vi "Create.vi"(7 "options":T13={"FIFO Options"={"Infinite Timeouts"=FALSE}, "Thread Options"={"Show FP On Call"=FALSE, "Close FP After Call"=FALSE, "Allow Debugging"=FALSE}, "Plugin Options"={"Default Components"=FALSE}, "Performance Options"={"Measure Period"=FALSE, "Measure Rx/Tx Duration"=FALSE}, "Data Server Options"={"Enable Data Server"=FALSE, "Period"=50}} {"Data Server Options"."Period" format="%d ms"}, 8 "error in (no error)":errorcluster, 11 "Device Item Ref":T19=18446744073709551615 format="%.0x") -> (0 "error out":errorcluster, 2 "framework configuration":T1, 3 "VeriStand Framework":refnum<class "VeriStand DSF.lvclass">)   [LabVIEW 2017, in "DSF Engine.lvlib" / "VeriStand DSF.lvclass"]
uses:
  VeriStand DSF.lvclass
  <vilib>/NI Veristand/Custom Device API/Custom Device Item Ref.ctl
  DSF Core.lvlibp/Classes/Framework/Framework Options.ctl
  DSF Core.lvlibp/Typedefs/DSF FIFO Options.ctl
  DSF Core.lvlibp/Classes/Thread/Thread Options.ctl
  DSF Core.lvlibp/Typedefs/DSF Plugin Options.ctl
  DSF Core.lvlibp/Typedefs/DSF Performance Options.ctl
  DSF Core.lvlibp/Classes/Framework/Data Server Options.ctl
  DSF Core.lvlibp/Typedefs/DSF Engine Framework Configuration.ctl
  DSF Core.lvlibp/Typedefs/DSF Engine Plugin Configuration.ctl
  DSF Core.lvlibp/Typedefs/DSF Timing Info.ctl
  DSF Core.lvlibp/Typedefs/DSF Engine Plugin Thread Configuration.ctl
  DSF Core.lvlibp/Typedefs/DSF Settings Info.ctl
  DSF Core.lvlibp/Typedefs/DSF Engine Transfer Group Configuration.ctl
  DSF Core.lvlibp/Typedefs/DSF Direction.ctl
  DSF Core.lvlibp/Typedefs/DSF Engine Transfer Configuration.ctl
  DSF Core.lvlibp/Typedefs/DSF Byte Order.ctl
  DSF Core.lvlibp/Typedefs/DSF Engine Channel Configuration.ctl
  DSF Core.lvlibp/Typedefs/DSF Data Type.ctl
  DSF Core.lvlibp/Typedefs/DSF Timeout Behavior.ctl
  VeriStand DSF.lvclass/VeriStand DSF.ctl
  Shared/DSF Shared.lvlib
  DSF Core.lvlibp/Classes/Configuration/Configuration Session.lvclass
  <vilib>/NI Veristand/Custom Device API/Custom Device API.lvlib
  DSF Core.lvlibp/Classes/Framework/Framework.lvclass
  DSF Core.lvlibp
  DSF Core.lvlibp/Classes/Thread/Thread.lvclass
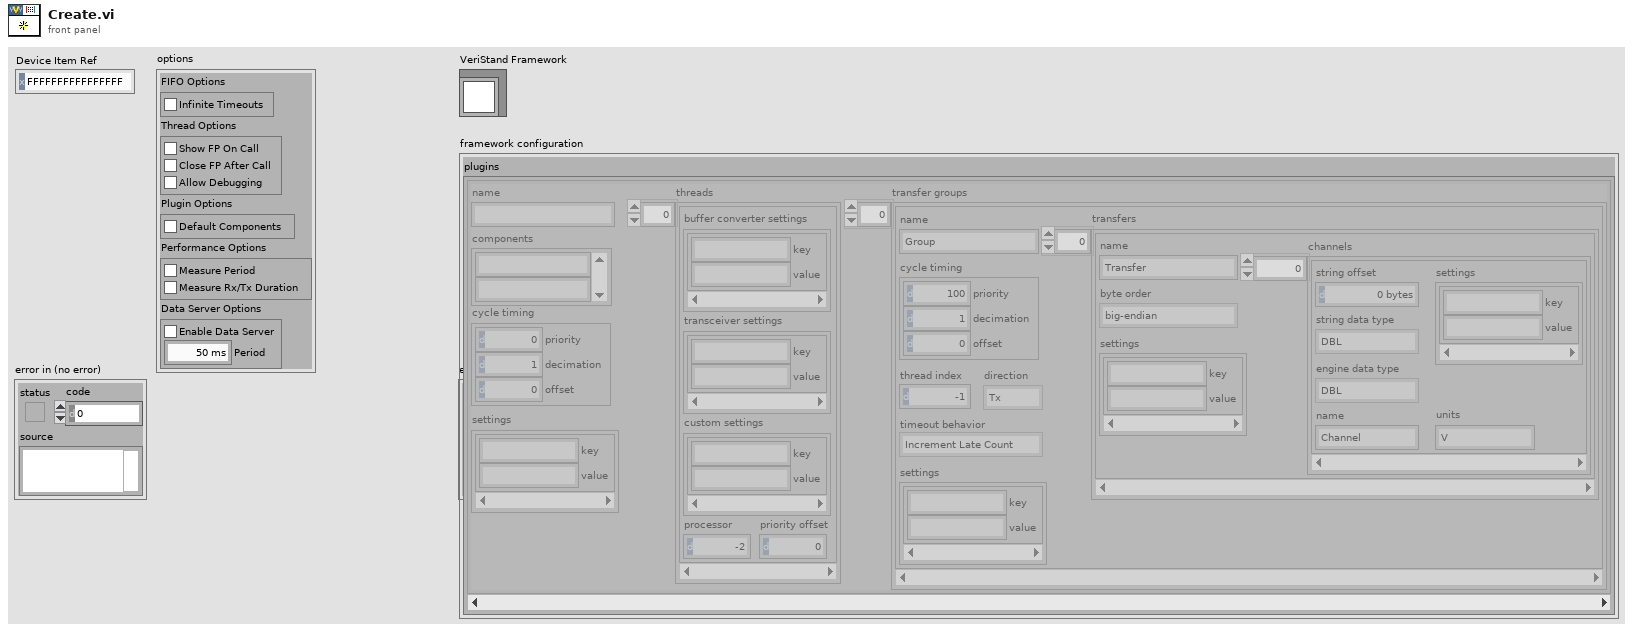
[diagram p1: front panel]
types:
  T1 = typedef "DSF Core.lvlibp/DSF Engine Framework Configuration.ctl" = cluster{"plugins":T2[]}
  T2 = typedef "DSF Core.lvlibp/DSF Engine Plugin Configuration.ctl" = cluster{"name":string, "components":string[], "cycle timing":T3, "threads":T4[], "transfer groups":T6[], "settings":T5}
  T3 = typedef "DSF Core.lvlibp/DSF Timing Info.ctl" = cluster{"priority":u64, "decimation":u64, "offset":u64}
  T4 = typedef "DSF Core.lvlibp/DSF Engine Plugin Thread Configuration.ctl" = cluster{"buffer converter settings":T5, "transceiver settings":T5, "custom settings":T5, "processor":i32, "priority offset":i16}
  T5 = typedef "DSF Core.lvlibp/DSF Settings Info.ctl" = cluster{"key":string, "value":string}[]
  T6 = typedef "DSF Core.lvlibp/DSF Engine Transfer Group Configuration.ctl" = cluster{"name":string, "direction":T7, "cycle timing":T3, "thread index":i32, "settings":T5, "transfers":T8[], "timeout behavior":T12}
  T7 = typedef "DSF Core.lvlibp/DSF Direction.ctl" = enum8{"Tx", "Rx"}
  T8 = typedef "DSF Core.lvlibp/DSF Engine Transfer Configuration.ctl" = cluster{"name":string, "byte order":T9, "settings":T5, "channels":T10[]}
  T9 = typedef "DSF Core.lvlibp/DSF Byte Order.ctl" = enum8{"big-endian", "little-endian"}
  T10 = typedef "DSF Core.lvlibp/DSF Engine Channel Configuration.ctl" = cluster{"string offset":u64, "string data type":T11, "engine data type":T11, "name":string, "settings":T5, "units":string}
  T11 = typedef "DSF Core.lvlibp/DSF Data Type.ctl" = enum8{"Bool", "SGL", "DBL", "I8", "I16", "I32", "I64", "U8", "U16", "U32", "U64"}
  T12 = typedef "DSF Core.lvlibp/DSF Timeout Behavior.ctl" = enum8{"Increment Late Count", "Throw Error"}
  T13 = typedef "DSF Core.lvlibp/Framework.lvclass/Framework Options.ctl" = cluster{"FIFO Options":T14, "Thread Options":T15, "Plugin Options":T16, "Performance Options":T17, "Data Server Options":T18}
  T14 = typedef "DSF Core.lvlibp/Framework.lvclass/DSF FIFO Options.ctl" = cluster{"Infinite Timeouts":bool}
  T15 = typedef "DSF Core.lvlibp/Thread.lvclass/Thread Options.ctl" = cluster{"Show FP On Call":bool, "Close FP After Call":bool, "Allow Debugging":bool}
  T16 = typedef "DSF Core.lvlibp/Framework.lvclass/DSF Plugin Options.ctl" = cluster{"Default Components":bool}
  T17 = typedef "DSF Core.lvlibp/DSF Performance Options.ctl" = cluster{"Measure Period":bool, "Measure Rx/Tx Duration":bool}
  T18 = typedef "DSF Core.lvlibp/Framework.lvclass/Data Server Options.ctl" = cluster{"Enable Data Server":bool, "Period":u32}
  T19 = typedef "Custom Device API.lvlib/Custom Device Item Ref.ctl" = u64
  T20 = enum16{"open", "replace", "create", "open or create", "replace or create", "replace or create with confirmation"}
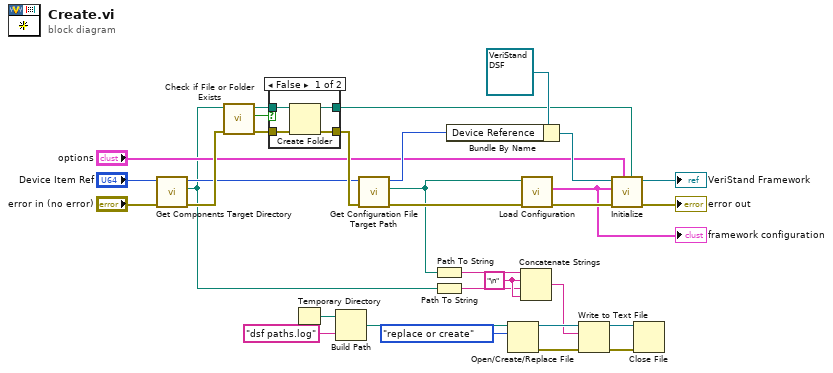
[diagram p0: block diagram]
diagram:
  w21 = "\n" ("string")
  n1 = call "Get Components Target Directory.vi"("error in (no error)"="error in (no error)", "Item Ref in"="Device Item Ref") -> ("error out"=w9:errorcluster, "components target directory"=w1:path, "Item Ref out"=w2:T19)  [unwired: 7 in]
  n2 = call <vilib>:"Check if File or Folder Exists.vi"("error in (no error)"=w9, "path"=w1) -> ("error out"=w8:errorcluster, "file or folder exists?"=w4:bool, "dup path"=w7:path)  [unwired: 7 in]
  n3 = case shown="False" w4 {
    tunnel: w8 -> [w36 w37]
    tunnel: [w35 w37] -> w5
    tunnel: w7 -> [w34 w38]
    tunnel: [w33 w38] -> w6
    frame False {
      n4 = Create Folder(path (use dialog)=w34, error in=w36) -> (created path=w33:path, error out=w35:errorcluster)  [unwired: 1 in, 1 out]
    }
    frame True {
    }
  }
  n5 = Temporary Directory() -> (w18:path)
  n6 = Build Path(base path=w18, name or relative path="dsf paths.log" ("file path (use dialog)")) -> (appended path=w16:path)
  n7 = call "Get Configuration File Target Path.vi"("error in (no error)"=w5, "Item Ref in"=w2) -> ("error out"=w14:errorcluster, "configuration target path"=w13:path, "Item Ref out"=w15:T19)  [unwired: 7 in]
  n8 = Path To String(path=w13) -> (string=w22:string)
  n9 = Path To String(path=w1) -> (string=w20:string)
  n10 = Bundle By Name(cluster=refnum<class "VeriStand DSF.lvclass"> refnum ("VeriStand Data Sharing Framework out"), "Device Reference"=w15) -> (w30:refnum<class "VeriStand DSF.lvclass">)
  n11 = Open/Create/Replace File(file path (use dialog)=w16, operation (0:open)=T20."replace or create") -> (refnum out=w26:refnum<file>, error out=w27:errorcluster)  [unwired: 4 in, 1 out]
  n12 = Concatenate Strings(w22, w21, w20, w21) -> (w19:string)
  n13 = call "Load Configuration.vi"("error in (no error)"=w14, "configuration file path"=w13) -> ("error out"=w31:errorcluster, "configuration"=w23:T1)  [unwired: 6 in, 2 out]
  "framework configuration" <- w23
  n14 = Write to Text File(file (use dialog)=w26, text=w19, error in=w27) -> (refnum out=w24:refnum<file>, error out=w25:errorcluster)  [unwired: 1 in, 1 out]
  n15 = call-dynamic "Initialize.vi"("components directory"=w6, "options"="options", "error in (no error)"=w31, "framework configuration"=w23, "VeriStand DSF in"=w30) -> ("error out"=→"error out":errorcluster, "VeriStand DSF out"=→"VeriStand Framework":refnum<class "VeriStand DSF.lvclass">)  [unwired: 5 in]
  n16 = Close File(refnum=w24, error in=w25) -> ()  [unwired: 2 out]
